vi "Pack4.vi"(8 "ClusterIn":T2={"Header size"=56, "MagicWord"=305419896, "byte order"=enum."little-endian", "Проверка конца пакета"=TRUE, "Проверка CRC8"=TRUE, "LastPacketIn"=6858, "MinimalString"=10000} {"MagicWord" format="%.0x"}, 11 "StringIn":string) -> (0 "ClusterOut":T1, 2 "Array":T3(array[cluster]) {"Reserve3" format="%08x"; "OverloadSamplesChannelY" format="%04x"; "OverloadSamplesChannelX" format="%04x"; "SamplingInterval" format="%#_6e"; "LoseSamples" format="%08x"; "EncodersParam2" format="%016x"; "EncodersParam1" format="%016x"; "CRC 8" format="%02x"; "Reserve2" format="%02x"; "Reserve" format="%02x"; "Ncycle" format="%04x"; "FrameFormatVersion" format="%02x"; "MagicWord" format="%.0x"}, 3 "StringLast":string)   [LabVIEW 2017]
uses:
  Control_EU/ClusterPack (Type).ctl
panel:
  out "PackRecived":bool
  out "PackSize":u32
  out "CheckCRC8":bool
  out "Header size":u32
  out "MWnotFund":bool
  out "MinStr":bool
  out "MinimalString":i32
  out "ErrorSizeCount":i32
  out "ErrorCRC8Count":i32
  out "ErrorCRC8":bool
  out "DataSize":u16
  out "RemainingBytes":u32
  out "OffsetMagicWord":i32
  out "DataSizeSmall":bool
  out "ErrorEndPack":bool
  out "ErrorSeqPackCount":i32
  out "ErrorSequence":bool
  out "LastPacket":u32
  out "PackGoodParsing":i32
  out "Iteration":i32
  out "MagicWordStr":string
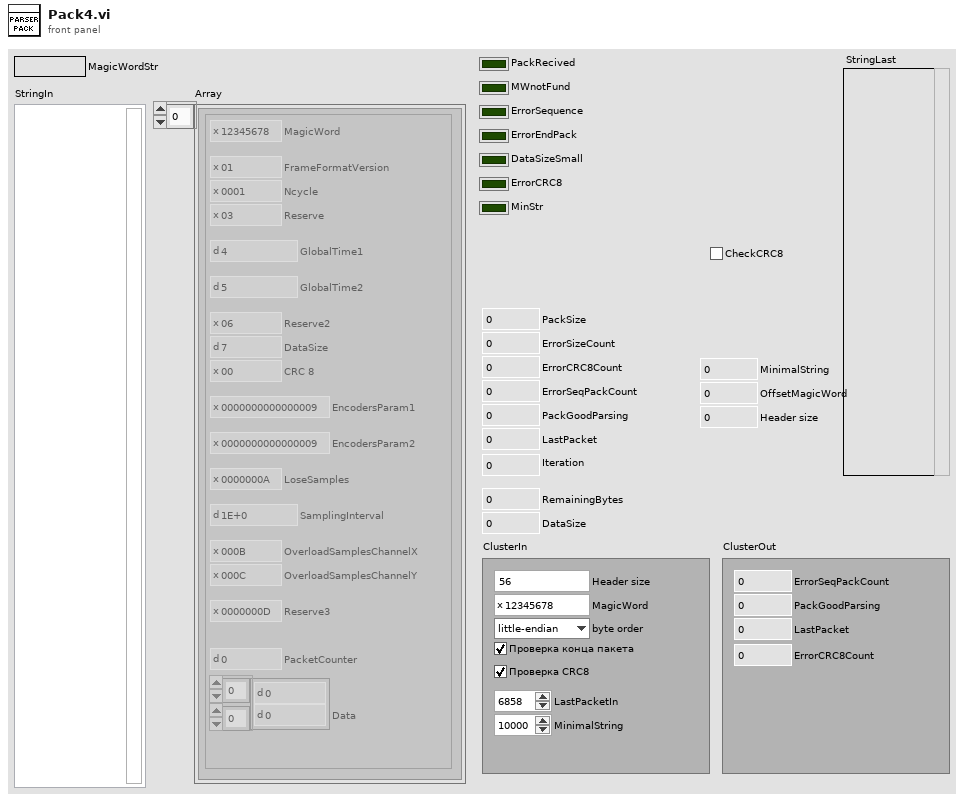
[diagram p1: front panel]
types:
  T1 = cluster{"PackGoodParsing":u32, "LastPacket":u32, "ErrorSeqPackCount":u32, "ErrorCRC8Count":u32}
  T2 = cluster{"Header size":u32, "MagicWord":u32, "byte order":enum16{"big-endian, network order", "native, host order", "little-endian"}, "Проверка конца пакета":bool, "Проверка CRC8":bool, "LastPacketIn":u32, "MinimalString":i32}
  T3 = cluster{"MagicWord":u32, "FrameFormatVersion":u8, "Ncycle":u16, "Reserve":u8, "GlobalTime1":u32, "GlobalTime2":u32, "Reserve2":u8, "DataSize":u16, "CRC 8":u8, "EncodersParam1":u64, "EncodersParam2":u64, "LoseSamples":u32, "SamplingInterval":sgl, "OverloadSamplesChannelX":u16, "OverloadSamplesChannelY":u16, "Reserve3":u32, "PacketCounter":u32, "Data":dbl[][]}[]
  T4 = typedef "ClusterPack (Type).ctl" = cluster{"MagicWord":u32, "FrameFormatVersion":u8, "Ncycle":u16, "Reserve":u8, "GlobalTime1":u32, "GlobalTime2":u32, "Reserve2":u8, "DataSize":u16, "CRC 8":u8, "EncodersParam1":u64, "EncodersParam2":u64, "LoseSamples":u32, "SamplingInterval":sgl, "OverloadSamplesChannelX":u16, "OverloadSamplesChannelY":u16, "Reserve3":u32, "PacketCounter":u32, "Data1":dbl[][]}
  T5 = enum16{"big-endian, network order", "native, host order", "little-endian"}
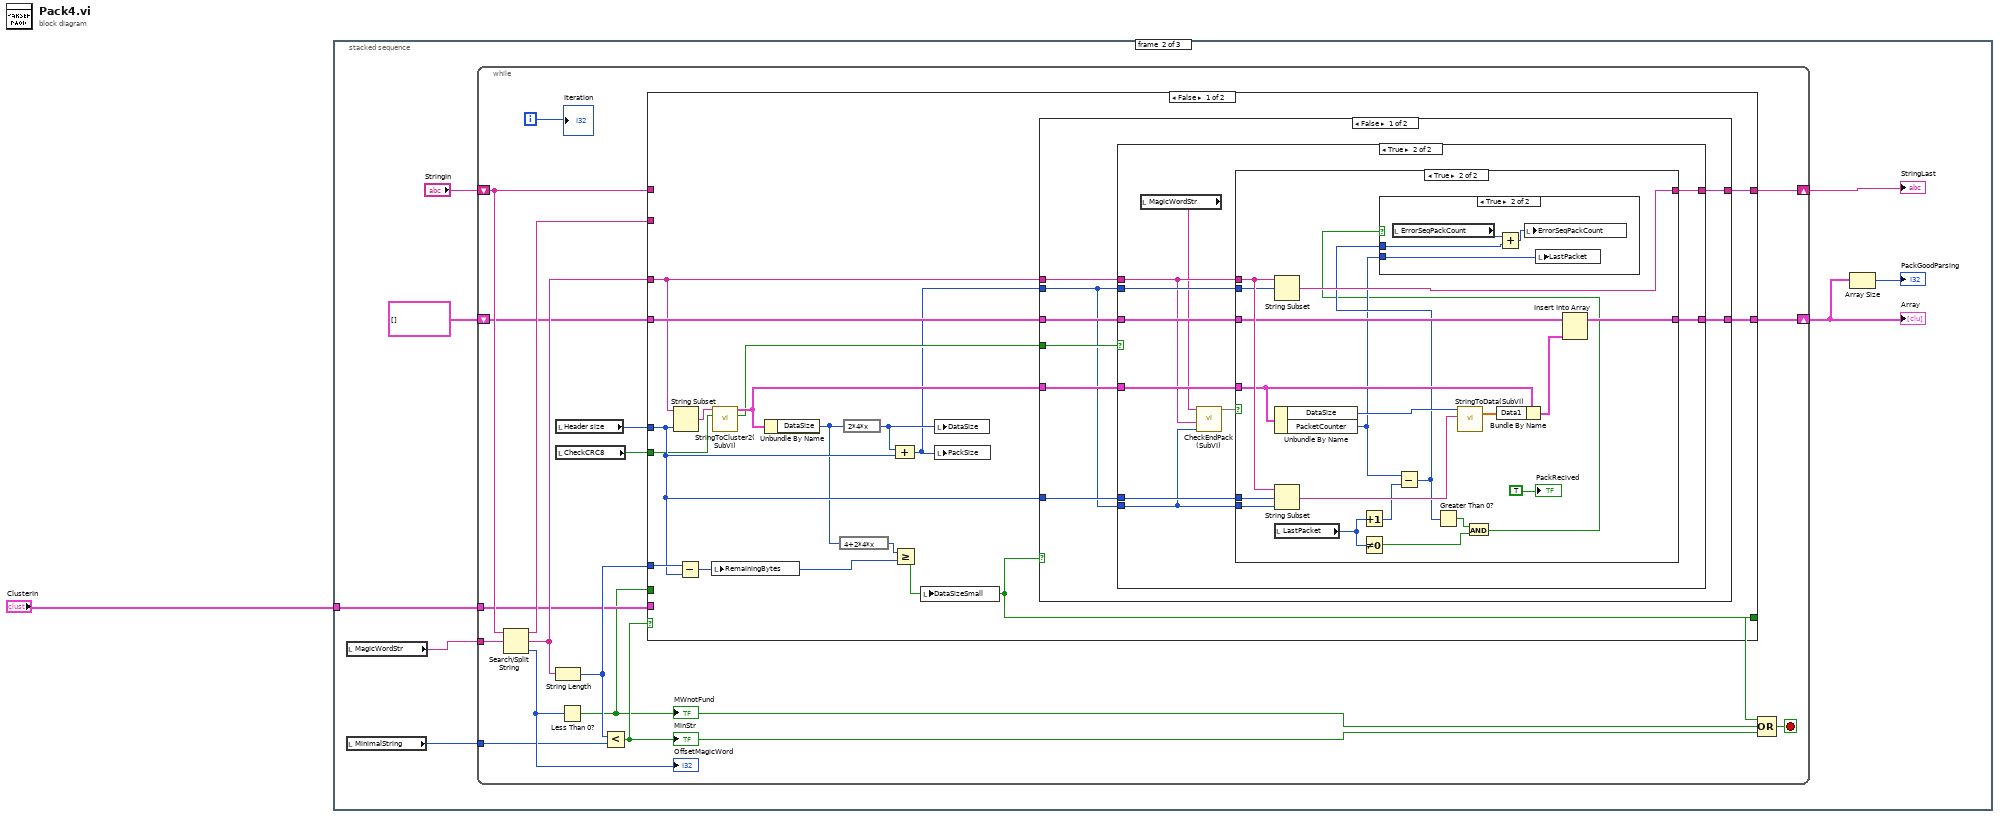
[diagram p0: block diagram]
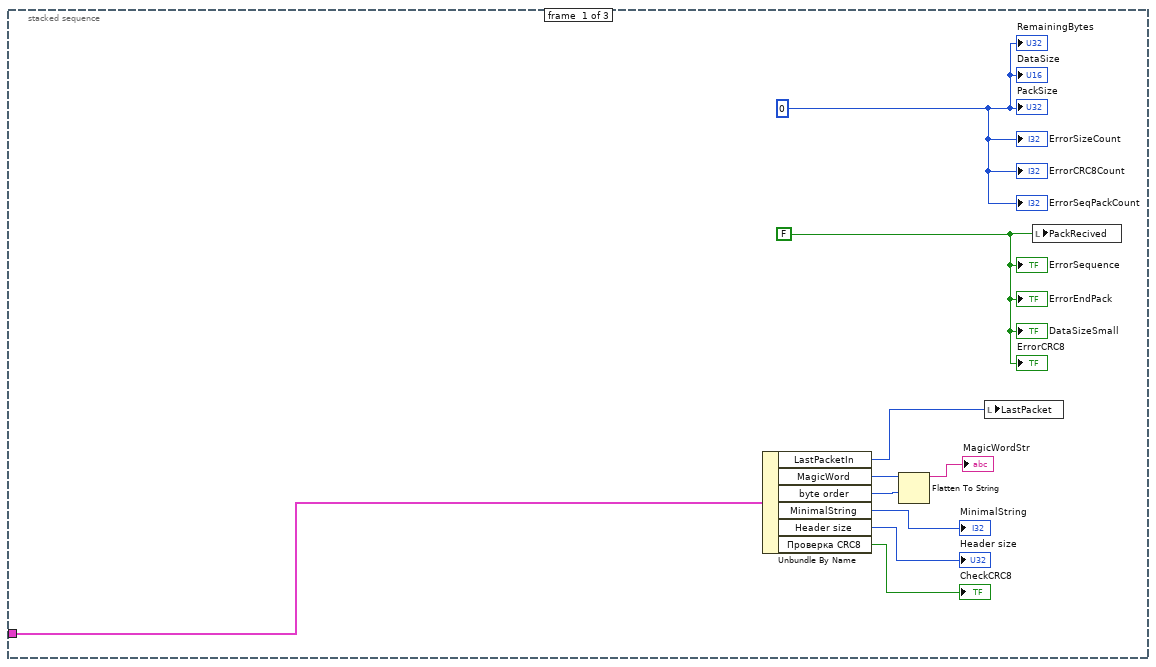
[diagram p2: hidden frame]
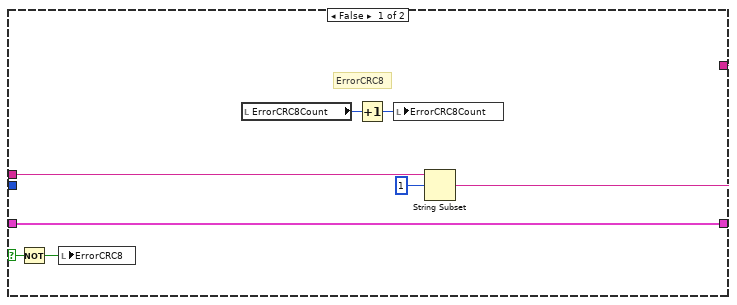
[diagram p3: hidden frame]
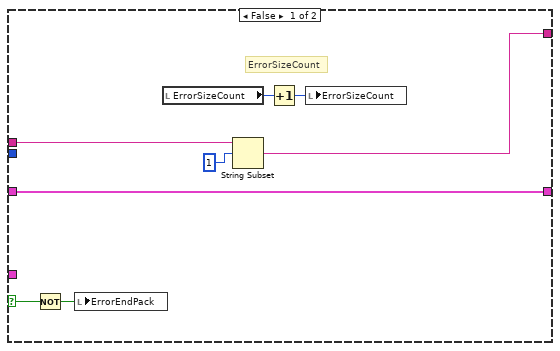
[diagram p4: hidden frame]
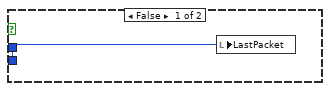
[diagram p5: hidden frame]
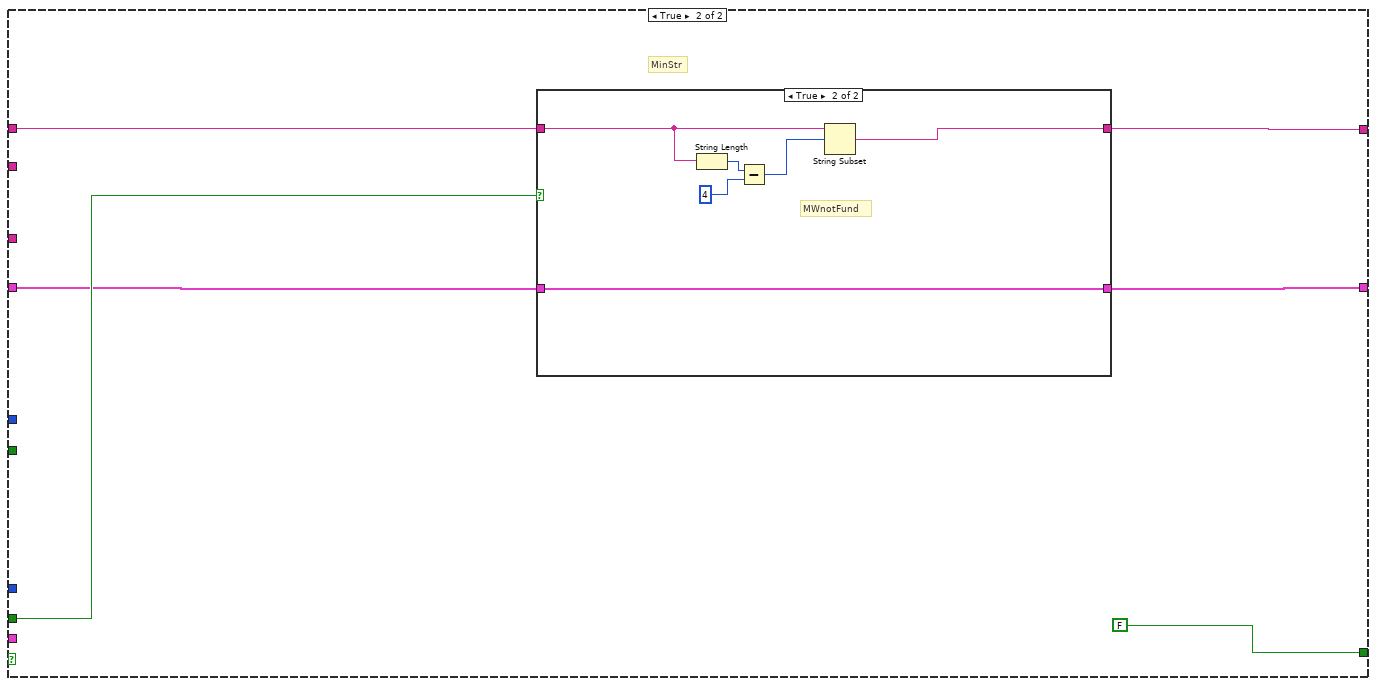
[diagram p7: hidden frame]
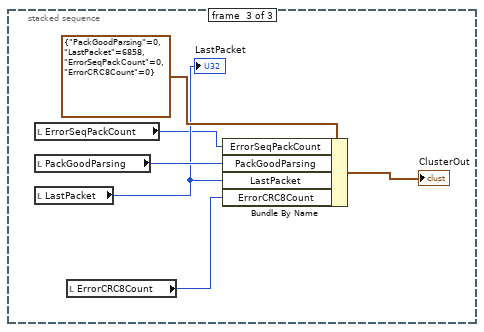
[diagram p9: hidden frame]
diagram:
  n1 = stacked-sequence {
    tunnel: "ClusterIn" -> [w6 w14 _]
    frame #0 {
      w3 = 0 ("ErrorSeqCount")
      w2 = FALSE ("PackLost")
      n2 = Unbundle By Name(w6) -> ("LastPacketIn"=w7:u32, "MagicWord"=w9:u32, "byte order"=w10:T5, "MinimalString"=→"MinimalString":i32, "Header size"=→"Header size":u32, "Проверка CRC8"=→"CheckCRC8":bool)
      n3 = Flatten To String(anything=w9, byte order (0:big-endian, network order)=w10) -> (data string=→"MagicWordStr":string)  [unwired: 2 in, 2 out]
      n4 = local write "LastPacket"(w7) -> ()
      n5 = local write "PackRecived"(w2) -> ()
      "ErrorSequence" <- w2
      "ErrorSeqPackCount" <- w3
      "ErrorEndPack" <- w2
      "ErrorCRC8Count" <- w3
      "DataSizeSmall" <- w2
      "ErrorSizeCount" <- w3
      "RemainingBytes" <- w3
      "DataSize" <- w3
      "PackSize" <- w3
      "ErrorCRC8" <- w2
    }
    frame #1 {
      n6 = local read "MagicWordStr"() -> (w12:string)
      n7 = local read "MinimalString"() -> (w13:i32)
      n8 = while {
        tunnel: w12 -> [w37]
        shift-right: [w25] -> w19
        shift-left: "StringIn" -> [w33]
        shift-right: [w29] -> w16
        shift-left: T4[] [] -> [w28]
        tunnel: w14 -> [w27]
        tunnel: w13 -> [w26]
        i -> [w30]
        stop <- w35 stop-if-true
        n9 = Search/Split String(string=w33, search string/char (-)=w37) -> (substring before match=w36:string, match + rest of string=w34:string, offset of match=w31:i32)  [unwired: 1 in]
        "OffsetMagicWord" <- w31
        n10 = local read "Header size"() -> (w21:u32)
        n11 = local read "CheckCRC8"() -> (w20:bool)
        n12 = String Length(string=w34) -> (length=w32:i32)
        n13 = Less Than 0?(x=w31) -> (x < 0?=w23:bool)
        "MWnotFund" <- w23
        n14 = Less?(x=w32, y=w26) -> (x < y?=w24:bool)
        "MinStr" <- w24
        n15 = case shown="False" w24 {
          tunnel: w34 -> [w44 _]
          tunnel: [w53 w117] -> w25
          tunnel: [w38 FALSE] -> w22
          tunnel: w36 -> [_ _]
          tunnel: w33 -> [_ w116]
          tunnel: w32 -> [w51 _]
          tunnel: w27 -> [_ _]
          tunnel: [w49 w119] -> w29
          tunnel: w28 -> [w48 w118]
          tunnel: w23 -> [_ w120]
          tunnel: w21 -> [w47 _]
          tunnel: w20 -> [w46 _]
          frame False {
            n16 = String Subset(string=w44, length (rest)=w47) -> (substring=w50:string)  [unwired: 1 in]
            n17 = Subtract(x=w51, y=w47) -> (x-y=w42:u32)
            n18 = local write "RemainingBytes"(w42) -> ()
            n19 = call "StringToCluster2(SubVI).vi"("Проверка CRC8"=w46, "StringIn"=w50) -> ("CRC8Good"=w40:bool, "ECC_Cluster"=w52:T4)  [unwired: 8 in]
            n20 = Unbundle By Name(w52) -> ("DataSize"=w45:u16)
            n21 = expression code="4+2*4*x"(w45) -> (w41:u16)
            n22 = expression code="2*4*x"(w45) -> (w43:u16)
            n23 = Greater Or Equal?(x=w41, y=w42) -> (x >= y?=w38:bool)
            n24 = Compound Arithmetic op=ADD(w43, w47) -> (w39:u32)
            n25 = local write "DataSizeSmall"(w38) -> ()
            n26 = local write "DataSize"(w43) -> ()
            n27 = local write "PackSize"(w39) -> ()
            n28 = case shown="False" w38 {
              tunnel: [w61 w113] -> w53
              tunnel: w52 -> [w60 _]
              tunnel: [w59 w114] -> w49
              tunnel: w48 -> [w58 w114]
              tunnel: w47 -> [w57 _]
              tunnel: w44 -> [w56 w113]
              tunnel: w40 -> [w55 _]
              tunnel: w39 -> [w54 _]
              frame False {
                n29 = case shown="True" w55 {
                  selector: w55 -> [w62 _]
                  tunnel: [w67 w79] -> w61
                  tunnel: w60 -> [_ w78]
                  tunnel: [w68 w77] -> w59
                  tunnel: w58 -> [w68 w76]
                  tunnel: w57 -> [_ w75]
                  tunnel: w54 -> [_ w74]
                  tunnel: w56 -> [w69 w73]
                  tunnel: w54 -> [_ w72]
                  frame False {
                    # "ErrorCRC8"
                    n30 = Not(x=w62) -> (.not. x?=w63:bool)
                    n31 = local write "ErrorCRC8"(w63) -> ()
                    n32 = local read "ErrorCRC8Count"() -> (w66:i32)
                    n33 = Increment(x=w66) -> (x+1=w65:i32)
                    n34 = local write "ErrorCRC8Count"(w65) -> ()
                    n35 = String Subset(string=w69, offset (0)=1) -> (substring=w67:string)  [unwired: 1 in]
                  }
                  frame True {
                    n36 = local read "MagicWordStr"() -> (w71:string)
                    n37 = call "CheckEndPack (SubVI).vi"("error in"=w72, "OfsetEndPack"=w73, "data"=w71) -> (3:w70)  [unwired: 5 in, 3 out]
                    n38 = case shown="True" w70 {
                      selector: w70 -> [w80 _]
                      tunnel: [w82 w107] -> w79
                      tunnel: w73 -> [w86 w106]
                      tunnel: w78 -> [_ w105]
                      tunnel: w72 -> [_ w104]
                      tunnel: w75 -> [_ w103]
                      tunnel: w74 -> [_ w102]
                      tunnel: [w87 w101] -> w77
                      tunnel: w76 -> [w87 w100]
                      frame False {
                        # "ErrorSizeCount"
                        n39 = Not(x=w80) -> (.not. x?=w81:bool)
                        n40 = local write "ErrorEndPack"(w81) -> ()
                        n41 = local read "ErrorSizeCount"() -> (w84:i32)
                        n42 = String Subset(string=w86, offset (0)=1) -> (substring=w82:string)  [unwired: 1 in]
                        n43 = Increment(x=w84) -> (x+1=w85:i32)
                        n44 = local write "ErrorSizeCount"(w85) -> ()
                      }
                      frame True {
                        n45 = String Subset(string=w106, offset (0)=w102) -> (substring=w107:string)  [unwired: 1 in]
                        n46 = Unbundle By Name(w105) -> ("DataSize"=w97:u16, "PacketCounter"=w93:u32)
                        n47 = String Subset(string=w106, offset (0)=w103, length (rest)=w104) -> (substring=w98:string)
                        n48 = local read "LastPacket"() -> (w90:u32)
                        n49 = Increment(x=w90) -> (x+1=w95:u32)
                        n50 = Not Equal To 0?(x=w90) -> (x != 0?=w89:bool)
                        n51 = Subtract(x=w93, y=w95) -> (x-y=w94:u32)
                        n52 = Greater Than 0?(x=w94) -> (x > 0?=w92:bool)
                        n53 = call "StringToData(SubVI).vi"("StringIn"=w98, "DataSize"=w97) -> ("DataOut"=w99:dbl[][])  [unwired: 9 in]
                        n54 = And(x=w92, y=w89) -> (x .and. y?=w91:bool)
                        n55 = case shown="True" w91 {
                          tunnel: w94 -> [_ w110]
                          tunnel: w93 -> [w108 w109]
                          frame False {
                            n56 = local write "LastPacket"(w108) -> ()
                          }
                          frame True {
                            n57 = local read "ErrorSeqPackCount"() -> (w112:i32)
                            n58 = Add(x=w112, y=w110) -> (x+y=w111:u32)
                            n59 = local write "ErrorSeqPackCount"(w111) -> ()
                            n60 = local write "LastPacket"(w109) -> ()
                          }
                        }
                        n61 = Bundle By Name(cluster=w105, "Data1"=w99) -> (w96:T4)
                        n62 = Insert Into Array(array=w100, new element=w96) -> (w101:T4[])  [unwired: 1 in]
                        "PackRecived" <- TRUE ("PackRecived")
                      }
                    }
                  }
                }
              }
              frame True {
              }
            }
          }
          frame True {
            # "MinStr"
            n63 = case shown="True" w120 {
              tunnel: [w121 w128] -> w119
              tunnel: w118 -> [w121 w128]
              tunnel: [w122 w123] -> w117
              tunnel: w116 -> [w122 w127]
              frame False {
                # "MWnotFund"
              }
              frame True {
                # "MWnotFund"
                n64 = String Length(string=w127) -> (length=w126:i32)
                n65 = Subtract(x=w126, y=4) -> (x-y=w124:i32)
                n66 = String Subset(string=w127, offset (0)=w124) -> (substring=w123:string)  [unwired: 1 in]
              }
            }
          }
        }
        n67 = Compound Arithmetic op=OR(w22, w23, w24) -> (w35:bool)
        "Iteration" <- w30
      }
      "StringLast" <- w19
      "Array" <- w16
      n68 = Array Size(array=w16) -> (size(s)=→"PackGoodParsing":i32)
    }
    frame #2 {
      n69 = local read "ErrorSeqPackCount"() -> (w130:i32)
      n70 = local read "PackGoodParsing"() -> (w132:i32)
      n71 = local read "LastPacket"() -> (w131:u32)
      "LastPacket" <- w131
      n72 = local read "ErrorCRC8Count"() -> (w129:i32)
      n73 = Bundle By Name(cluster=T1 {"PackGoodParsing"=0, "LastPacket"=6858, "ErrorSeqPackCount"=0, "ErrorCRC8Count"=0} ("ClusterOut"), "ErrorSeqPackCount"=w130, "PackGoodParsing"=w132, "LastPacket"=w131, "ErrorCRC8Count"=w129) -> (→"ClusterOut":T1)
    }
  }
